vi "initialize.vi"(8 "error in (no error)":errorcluster, 9 "Baudrate":dbl, 10 "COM Port":refnum<visa-resource-name>, 11 "Controller in":refnum<class "Controller.lvclass">) -> (0 "error out":errorcluster, 3 "Controller out":refnum<class "Controller.lvclass">)   [LabVIEW 2019, in "Controller.lvclass"]
uses:
  Controller.lvclass
  Controller.lvclass/Controller.ctl
  Communication/Communication.lvclass
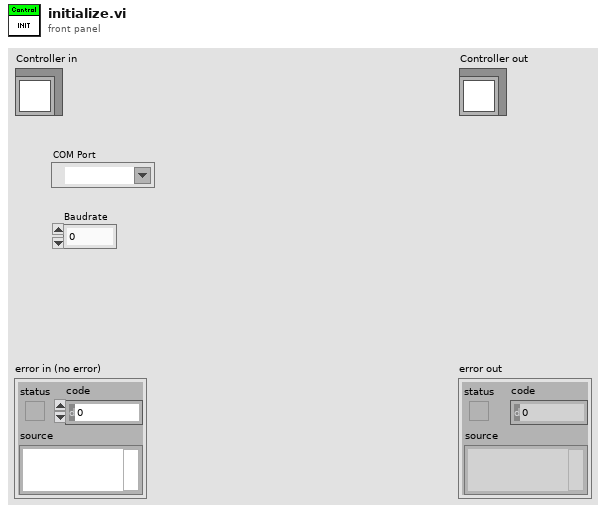
[diagram p1: front panel]
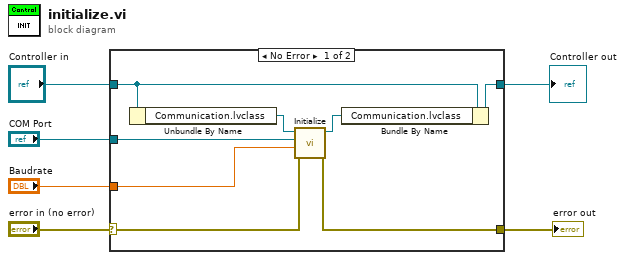
[diagram p0: block diagram]
diagram:
  n1 = case shown="No Error" "error in (no error)" {
    selector: "error in (no error)" -> [w8 w16]
    tunnel: [w9 w16] -> w5
    tunnel: [w10 w15] -> w3
    tunnel: "Controller in" -> [w11 w15]
    tunnel: "COM Port" -> [w12 _]
    tunnel: "Baudrate" -> [w7 _]
    frame No Error {
      n2 = Unbundle By Name(w11) -> ("Communication.lvclass"=w14:refnum<class "Communication.lvclass">)
      n3 = call-dynamic "Initialize.vi"("error in (no error)"=w8, "Baudrate"=w7, "COM Port"=w12, "Communication in"=w14) -> ("error out"=w9:errorcluster, "Communication out"=w13:refnum<class "Communication.lvclass">)  [unwired: 6 in]
      n4 = Bundle By Name(cluster=w11, "Communication.lvclass"=w13) -> (w10:refnum<class "Controller.lvclass">)
    }
    frame Error {
    }
  }
  "error out" <- w5
  "Controller out" <- w3
